vi "Post (NT Enum (Index & Choices)).vi"(6 "timestamp in":timestamp, 7 "PV name":string, 8 "error in (no error)":errorcluster, 9 "choices in":string[](array[string]), 10 "index in":u16, 11 "Server in":refnum<class "Server.lvclass">) -> (0 "error out":errorcluster, 1 "choices out":string[](array[string]), 2 "index out":u16, 3 "Server out":refnum<class "Server.lvclass">, 4 "timestamp out":timestamp)   [LabVIEW 2020, in "PV Access.lvlib" / "PVA Server.lvlib" / "Server.lvclass"]
doc: "If you just want to set the index, leave the <B>choices in</B> control unset. Only array containg at least one element will be used."
uses:
  Server.lvclass
  PV Data/PV Data/PV Data.lvclass
  Source/Source.lvclass
  Server.lvclass/Server.ctl
  PV Data/PV Data/Write Field (I32).vi
  PV Data/PV Data/Write Field (String Array).vi
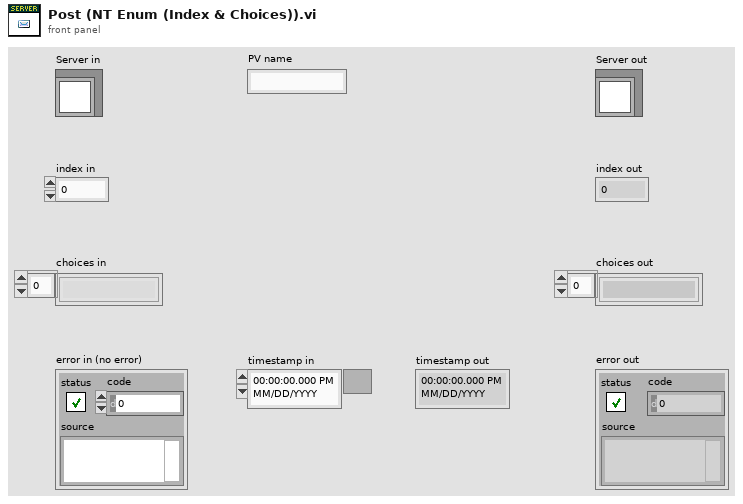
[diagram p1: front panel]
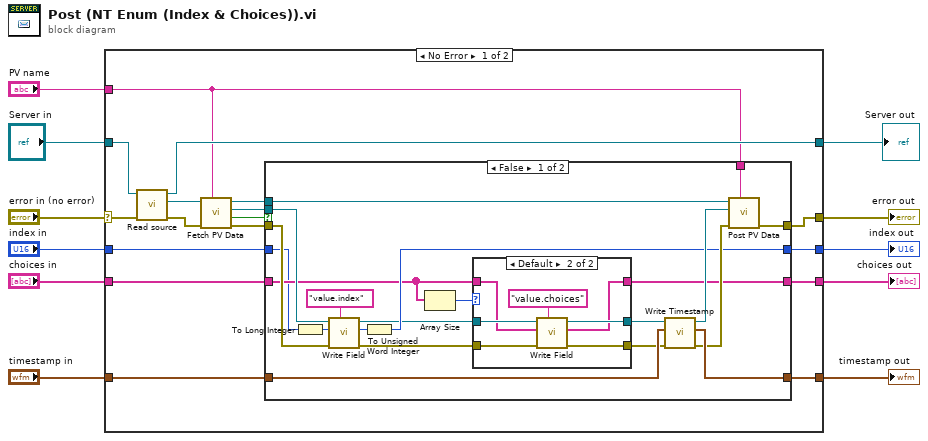
[diagram p0: block diagram]
diagram:
  n1 = case shown="No Error" "error in (no error)" {
    selector: "error in (no error)" -> [w26 w68]
    tunnel: [w18 w68] -> w5
    tunnel: [w27 w67] -> w3
    tunnel: "Server in" -> [w28 w67]
    tunnel: "PV name" -> [w19 _]
    tunnel: "index in" -> [w17 w66]
    tunnel: [w16 w66] -> w6
    tunnel: "timestamp in" -> [w22 w65]
    tunnel: [w21 w65] -> w4
    tunnel: "choices in" -> [w14 w64]
    tunnel: [w15 w64] -> w1
    frame No Error {
      n2 = call "Read source.vi"("error in (no error)"=w26, "Server in"=w28) -> ("error out"=w24:errorcluster, "Source"=w25:refnum<class "Source.lvclass">, "Server out"=w27:refnum<class "Server.lvclass">)  [unwired: 7 in]
      n3 = call "Fetch PV Data.vi"("PV name"=w19, "error in"=w24, "Source in"=w25) -> ("error out"=w12:errorcluster, "PV not found?"=w13:bool, "PV Data out"=w23:refnum<class "PV Data.lvclass">, "Source out"=w20:refnum<class "Source.lvclass">)  [unwired: 5 in]
      n4 = case shown="False" w13 {
        tunnel: w17 -> [w30 w60]
        tunnel: w23 -> [w49 _]
        tunnel: w12 -> [w48 w62]
        tunnel: w22 -> [w46 w63]
        tunnel: [w45 w63] -> w21
        tunnel: w20 -> [w42 _]
        tunnel: w19 -> [w41 _]
        tunnel: [w40 w62] -> w18
        tunnel: [w38 w60] -> w16
        tunnel: [w33 w61] -> w15
        tunnel: w14 -> [w31 w61]
        frame False {
          n5 = To Long Integer(number=w30) -> (32bit integer=w29:i32)
          n6 = call-poly "Write Field.vi"("field name"="value.index", "error in"=w48, "value"=w29, "PV Data in"=w49) -> ("error out"=w36:errorcluster, "value out"=w39:i32, "PV Data out"=w37:refnum<class "PV Data.lvclass">)  [unwired: 5 in]
          n7 = To Unsigned Word Integer(number=w39) -> (unsigned 16bit integer=w38:u16)
          n8 = Array Size(array=w31) -> (size(s)=w32:i32)
          n9 = case shown="Default" w32 {
            tunnel: w37 -> [w51 w58]
            tunnel: w36 -> [w50 w57]
            tunnel: [w50 w56] -> w35
            tunnel: [w51 w55] -> w34
            tunnel: w31 -> [w52 w54]
            tunnel: [w52 w53] -> w33
            frame 0 {
            }
            frame Default {
              n10 = call-poly "Write Field.vi"("field name"="value.choices", "error in"=w57, "value"=w54, "PV Data in"=w58) -> ("error out"=w56:errorcluster, "value out"=w53:string[], "PV Data out"=w55:refnum<class "PV Data.lvclass">)  [unwired: 5 in]
            }
          }
          n11 = call "Write Timestamp.vi"("error in"=w35, "timestamp in"=w46, "PV Data in"=w34) -> ("error out"=w44:errorcluster, "timestamp out"=w45:timestamp, "PV Data out"=w43:refnum<class "PV Data.lvclass">)  [unwired: 5 in, 1 out]
          n12 = call "Post PV Data.vi"("PV name"=w41, "error in"=w44, "PV Data in"=w43, "Source in"=w42) -> ("error out"=w40:errorcluster)  [unwired: 6 in, 1 out]
        }
        frame True {
        }
      }
    }
    frame Error {
    }
  }
  "error out" <- w5
  "Server out" <- w3
  "index out" <- w6
  "timestamp out" <- w4
  "choices out" <- w1
